vi "pl1000CloseUnit.vi"(8 "error in (no error)":errorcluster, 11 "pl1000 handle":i16) -> (0 "error out":errorcluster, 3 "pl1000 handle out":i16)   [LabVIEW 2016, in "pl1000.lvlib"]
uses:
  pl1000.lvlib
  pl1000.dll
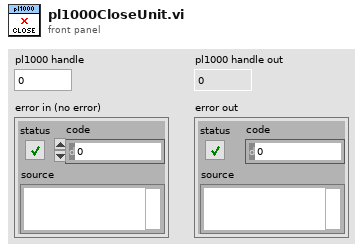
[diagram p1: front panel]
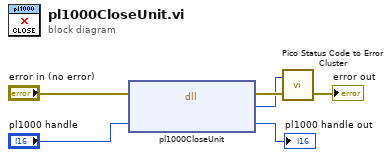
[diagram p0: block diagram]
diagram:
  n1 = dll-call lib="pl1000.dll" fn="pl1000CloseUnit"(error in="error in (no error)", "handle"="pl1000 handle") -> (error out=w5:errorcluster, "status"=w4:u32, "handle"=→"pl1000 handle out":i16)  [unwired: 2 in, 1 out]
  n2 = call "Pico Status Code to Error Cluster.vi"("error in"=w5, "PICO_STATUS"=w4) -> ("error out"=→"error out":errorcluster)  [unwired: 1 in]
